vi "Robot Arm Drawbridge.vi"(7 "Motor Speed":dbl, 8 "Abort":bool, 9 "Start Drawbridge":bool, 10 "Limit Switch Shoulder":bool, 11 "Limit Switch Elbow":bool) -> (0 "Done":bool, 1 "Arcada Drive":T1, 2 "Set Shoulder":dbl, 3 "Set Elbow":dbl)   [LabVIEW 2015]
uses:
  drawbride_auto_state.ctl
  Sensors.vi
panel:
  in  "Time Target (s)":dbl=1.0
  in  "Drive Time":dbl
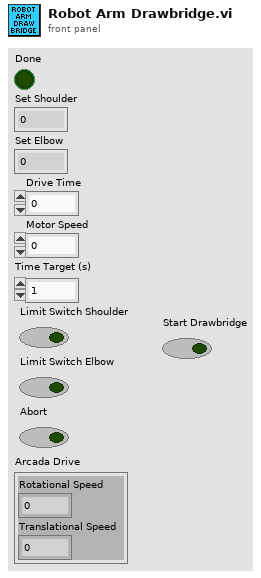
[diagram p1: front panel]
types:
  T1 = cluster{"Rotational Speed":dbl, "Translational Speed":dbl}
  T2 = typedef "drawbride_auto_state.ctl" = enum16{"Ready", "Arm up over gate", "Hook arm", "Arm Down", "Drive over Gate", "Arm to rest", "Stop"}
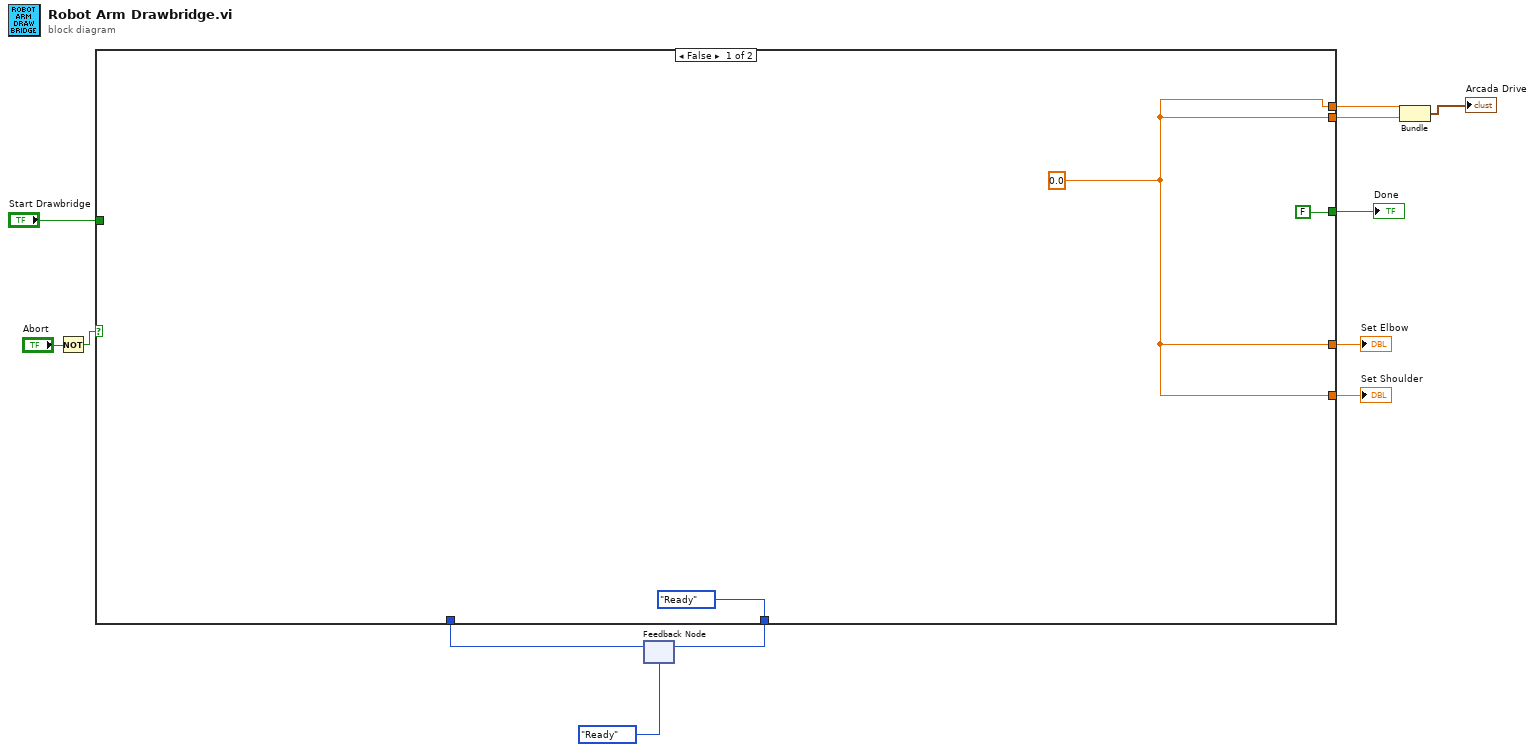
[diagram p0: block diagram]
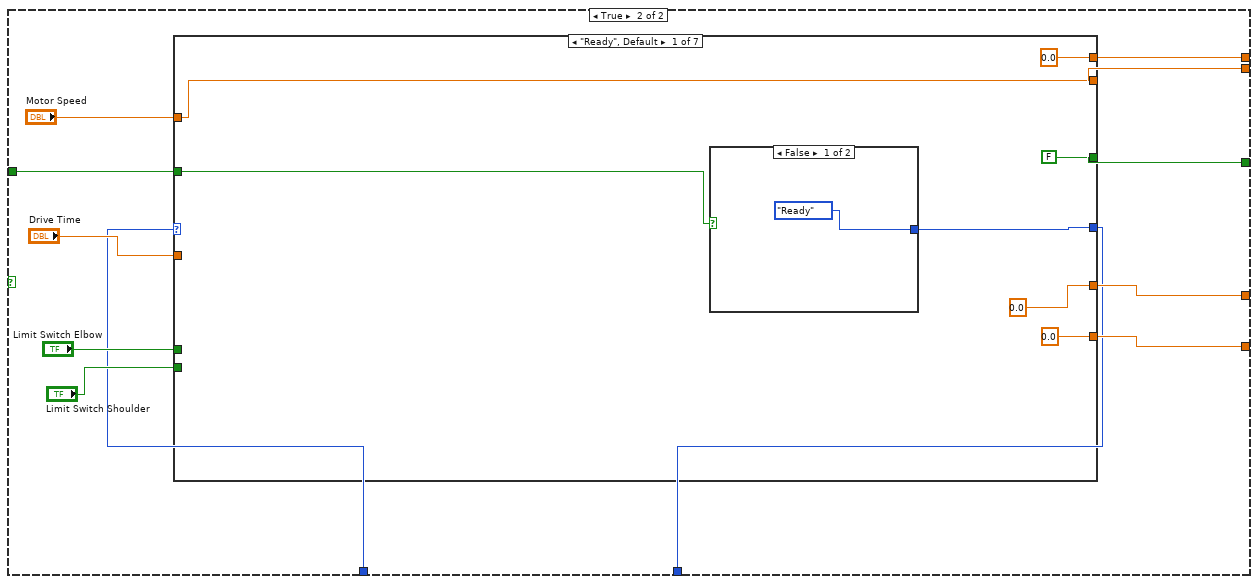
[diagram p2: hidden frame]
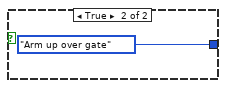
[diagram p3: hidden frame]
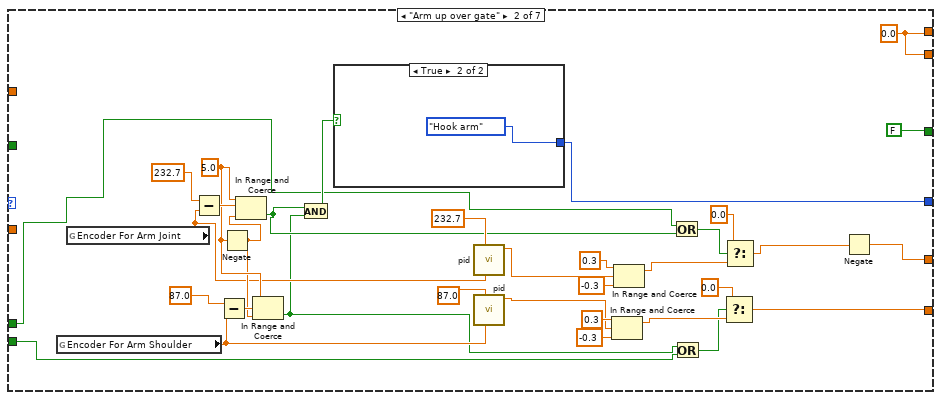
[diagram p4: hidden frame]
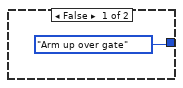
[diagram p5: hidden frame]
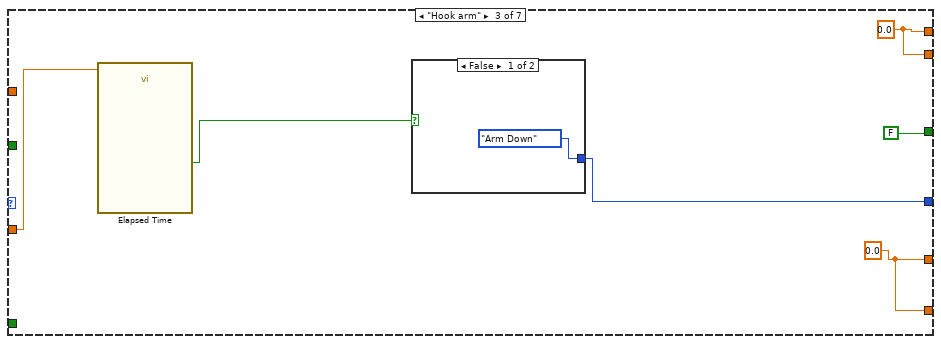
[diagram p6: hidden frame]
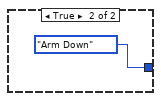
[diagram p7: hidden frame]
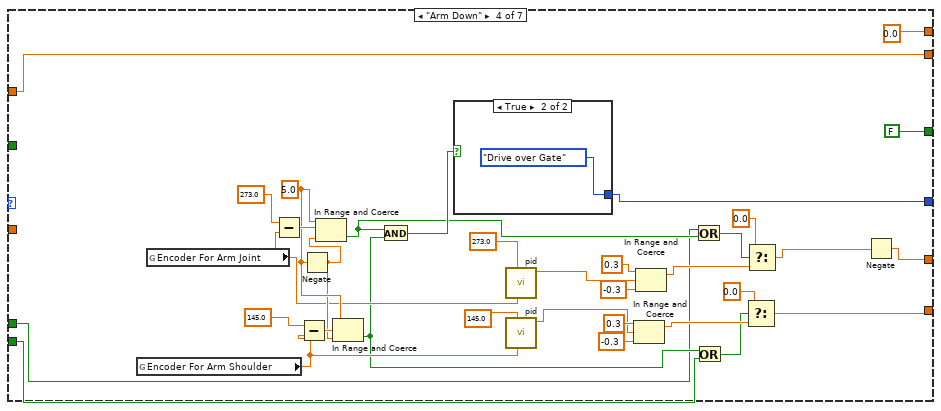
[diagram p8: hidden frame]
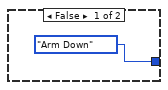
[diagram p9: hidden frame]
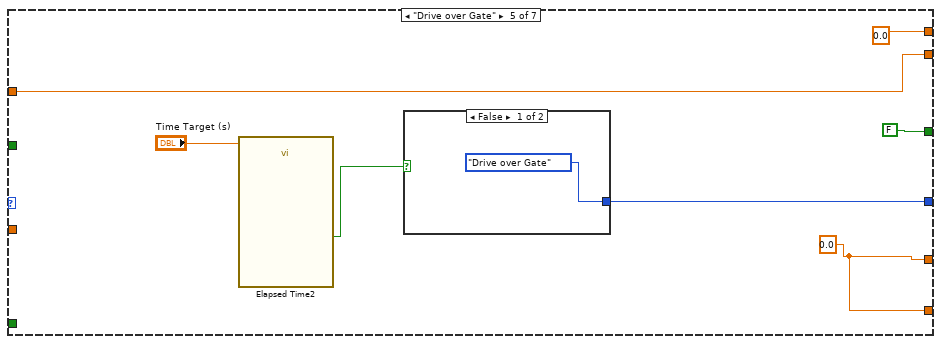
[diagram p10: hidden frame]
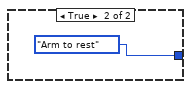
[diagram p11: hidden frame]
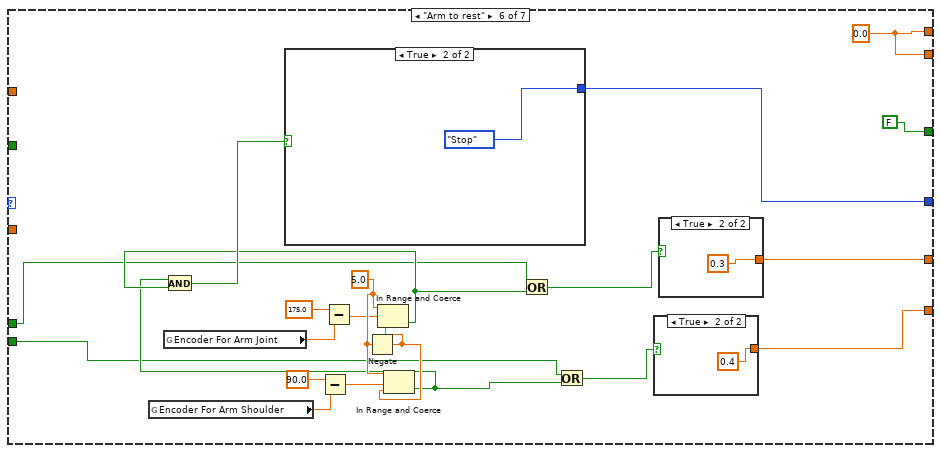
[diagram p12: hidden frame]
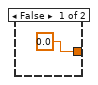
[diagram p13: hidden frame]
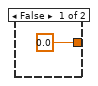
[diagram p14: hidden frame]
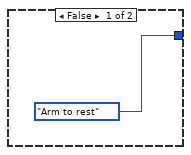
[diagram p15: hidden frame]
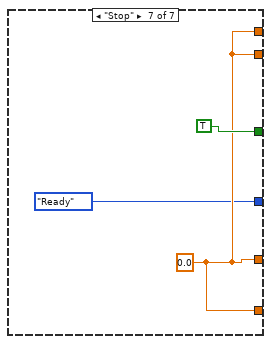
[diagram p16: hidden frame]
diagram:
  n1 = Not(x="Abort") -> (.not. x?=w5:bool)
  n2 = feedback #1(drawbride_auto_state."Ready") -> (w2:T2)
  n3 = case shown="False" w5 {
    tunnel: [w15 w23] -> w12
    tunnel: [w15 w22] -> w11
    tunnel: [FALSE w21] -> w9
    tunnel: [w15 w20] -> w8
    tunnel: [w15 w19] -> w7
    tunnel: "Start Drawbridge" -> [_ w18]
    tunnel: w2 -> [_ w17]
    tunnel: [drawbride_auto_state."Ready" w16] -> w1
    frame False {
      w15 = 0.0
    }
    frame True {
      n4 = case shown="\"Ready\", Default" w17 {
        tunnel: "Motor Speed" -> [w34 _ _ w113 w122 _ _]
        tunnel: "Drive Time" -> [_ _ w75 _ _ _ _]
        tunnel: [0.0 w57 w76 0.0 0.0 w143 w152] -> w23
        tunnel: [FALSE FALSE FALSE FALSE FALSE FALSE TRUE] -> w21
        tunnel: [0.0 ("Set Motor at S") w41 w73 w84 w116 w139 w152] -> w20
        tunnel: [0.0 ("Set Motor at 1") w42 w73 w85 w116 w140 w152] -> w19
        tunnel: [w34 w57 w76 w113 w122 w143 w152] -> w22
        tunnel: "Limit Switch Shoulder" -> [_ w37 _ w82 _ w125 _]
        tunnel: "Limit Switch Elbow" -> [_ w40 _ w80 _ w126 _]
        tunnel: [w29 w56 w72 w100 w117 w141 drawbride_auto_state."Ready"] -> w16
        tunnel: w18 -> [w28 _ _ _ _ _ _]
        frame "Ready", Default {
          n5 = case shown="False" w28 {
            tunnel: [drawbride_auto_state."Ready" drawbride_auto_state."Arm up over gate"] -> w29
            frame False {
            }
            frame True {
            }
          }
        }
        frame "Arm up over gate" {
          w61 = 5.0
          w57 = 0.0
          n6 = global read "Sensors.vi" "Encoder For Arm Shoulder"() -> (w59:dbl)
          n7 = global read "Sensors.vi" "Encoder For Arm Joint"() -> (w58:dbl)
          n8 = Subtract(x=232.7 ("setpoint"), y=w58) -> (x-y=w63:dbl)
          n9 = Subtract(x=87.0 ("setpoint"), y=w59) -> (x-y=w66:dbl)
          n10 = Negate(x=w61) -> (-x=w60:dbl)
          n11 = In Range and Coerce(upper limit=w61, x=w63, lower limit=w60) -> (In Range?=w39:bool)  [unwired: 1 out]
          n12 = In Range and Coerce(upper limit=w61, x=w66, lower limit=w60) -> (In Range?=w38:bool)  [unwired: 1 out]
          n13 = And(x=w39, y=w38) -> (x .and. y?=w64:bool)
          n14 = case shown="True" w64 {
            tunnel: [drawbride_auto_state."Arm up over gate" drawbride_auto_state."Hook arm"] -> w56
            frame False {
            }
            frame True {
            }
          }
          n15 = call "pid.vi"("y"=w58, "setpoint"=232.7) -> ("Motor Command"=w44:dbl)  [unwired: 9 in]
          n16 = call "pid.vi"("y"=w59, "setpoint"=87.0) -> ("Motor Command"=w43:dbl)  [unwired: 9 in]
          n17 = In Range and Coerce(upper limit=0.3, x=w43, lower limit=-0.3) -> (coerced(x)=w54:dbl)  [unwired: 1 out]
          n18 = In Range and Coerce(upper limit=0.3, x=w44, lower limit=-0.3) -> (coerced(x)=w55:dbl)  [unwired: 1 out]
          n19 = Or(x=w40, y=w39) -> (x .or. y?=w50:bool)
          n20 = Or(x=w38, y=w37) -> (x .or. y?=w51:bool)
          n21 = Select(t=0.0, s=w51, f=w54) -> (s? t:f=w42:dbl)
          n22 = Select(t=0.0, s=w50, f=w55) -> (s? t:f=w45:dbl)
          n23 = Negate(x=w45) -> (-x=w41:dbl)
        }
        frame "Hook arm" {
          w73 = 0.0
          w76 = 0.0
          n24 = call "Elapsed Time"("Time Target (s)"=w75) -> ("Time has Elapsed"=w74:bool)  [unwired: 11 in, 7 out]
          n25 = case shown="False" w74 {
            tunnel: [drawbride_auto_state."Arm Down" drawbride_auto_state."Arm Down"] -> w72
            frame False {
            }
            frame True {
            }
          }
        }
        frame "Arm Down" {
          w106 = 5.0
          n26 = global read "Sensors.vi" "Encoder For Arm Shoulder"() -> (w99:dbl)
          n27 = global read "Sensors.vi" "Encoder For Arm Joint"() -> (w102:dbl)
          n28 = Subtract(x=273.0 ("setpoint"), y=w102) -> (x-y=w108:dbl)
          n29 = Subtract(x=145.0 ("setpoint"), y=w99) -> (x-y=w110:dbl)
          n30 = Negate(x=w106) -> (-x=w105:dbl)
          n31 = In Range and Coerce(upper limit=w106, x=w108, lower limit=w105) -> (In Range?=w81:bool)  [unwired: 1 out]
          n32 = In Range and Coerce(upper limit=w106, x=w110, lower limit=w105) -> (In Range?=w83:bool)  [unwired: 1 out]
          n33 = And(x=w81, y=w83) -> (x .and. y?=w101:bool)
          n34 = case shown="True" w101 {
            tunnel: [drawbride_auto_state."Arm Down" drawbride_auto_state."Drive over Gate"] -> w100
            frame False {
            }
            frame True {
            }
          }
          n35 = call "pid.vi"("y"=w102, "setpoint"=273.0) -> ("Motor Command"=w87:dbl)  [unwired: 9 in]
          n36 = call "pid.vi"("y"=w99, "setpoint"=145.0) -> ("Motor Command"=w86:dbl)  [unwired: 9 in]
          n37 = In Range and Coerce(upper limit=0.3, x=w86, lower limit=-0.3) -> (coerced(x)=w97:dbl)  [unwired: 1 out]
          n38 = In Range and Coerce(upper limit=0.3, x=w87, lower limit=-0.3) -> (coerced(x)=w98:dbl)  [unwired: 1 out]
          n39 = Or(x=w80, y=w81) -> (x .or. y?=w93:bool)
          n40 = Or(x=w83, y=w82) -> (x .or. y?=w94:bool)
          n41 = Select(t=0.0, s=w94, f=w97) -> (s? t:f=w85:dbl)
          n42 = Select(t=0.0, s=w93, f=w98) -> (s? t:f=w88:dbl)
          n43 = Negate(x=w88) -> (-x=w84:dbl)
        }
        frame "Drive over Gate" {
          w116 = 0.0
          n44 = call "Elapsed Time2"("Time Target (s)"="Time Target (s)") -> ("Time has Elapsed"=w118:bool)  [unwired: 11 in, 7 out]
          n45 = case shown="False" w118 {
            tunnel: [drawbride_auto_state."Drive over Gate" drawbride_auto_state."Arm to rest"] -> w117
            frame False {
            }
            frame True {
            }
          }
        }
        frame "Arm to rest" {
          w137 = 5.0
          w143 = 0.0
          n46 = global read "Sensors.vi" "Encoder For Arm Shoulder"() -> (w133:dbl)
          n47 = global read "Sensors.vi" "Encoder For Arm Joint"() -> (w132:dbl)
          n48 = Subtract(x=90.0, y=w133) -> (x-y=w136:dbl)
          n49 = Subtract(x=175.0, y=w132) -> (x-y=w135:dbl)
          n50 = Negate(x=w137) -> (-x=w138:dbl)
          n51 = In Range and Coerce(upper limit=w137, x=w135, lower limit=w138) -> (In Range?=w128:bool)  [unwired: 1 out]
          n52 = In Range and Coerce(upper limit=w137, x=w136, lower limit=w138) -> (In Range?=w127:bool)  [unwired: 1 out]
          n53 = And(x=w127, y=w128) -> (x .and. y?=w142:bool)
          n54 = case shown="True" w142 {
            tunnel: [drawbride_auto_state."Arm to rest" drawbride_auto_state."Stop"] -> w141
            frame False {
            }
            frame True {
            }
          }
          n55 = Or(x=w126, y=w128) -> (x .or. y?=w129:bool)
          n56 = Or(x=w125, y=w127) -> (x .or. y?=w130:bool)
          n57 = case shown="True" w130 {
            tunnel: [0.0 0.4] -> w140
            frame False {
            }
            frame True {
            }
          }
          n58 = case shown="True" w129 {
            tunnel: [0.0 0.3] -> w139
            frame False {
            }
            frame True {
            }
          }
        }
        frame "Stop" {
          w152 = 0.0
        }
      }
    }
  }
  "Done" <- w9
  "Set Elbow" <- w8
  "Set Shoulder" <- w7
  n59 = feedback-in #1(w1) -> ()
  n60 = Bundle(w12, "Motor Speed"=w11) -> (→"Arcada Drive":cluster{dbl, "Motor Speed":dbl})  [unwired: 1 in]
